vi "ScriptLoop.vi"   [LabVIEW 2012]
types:
  T1 = cluster{"Name":string, "Parameters":string[], "Start Conditional":cluster{"String":string, "avgs":cluster{"Expression":string, "Durration":dbl, "Replacement":string, "Values":dbl[]}[]}, "End Conditional":cluster{"String":string, "avgs":cluster{"Expression":string, "Durration":dbl, "Replacement":string, "Values":dbl[]}[]}, "Running":bool}
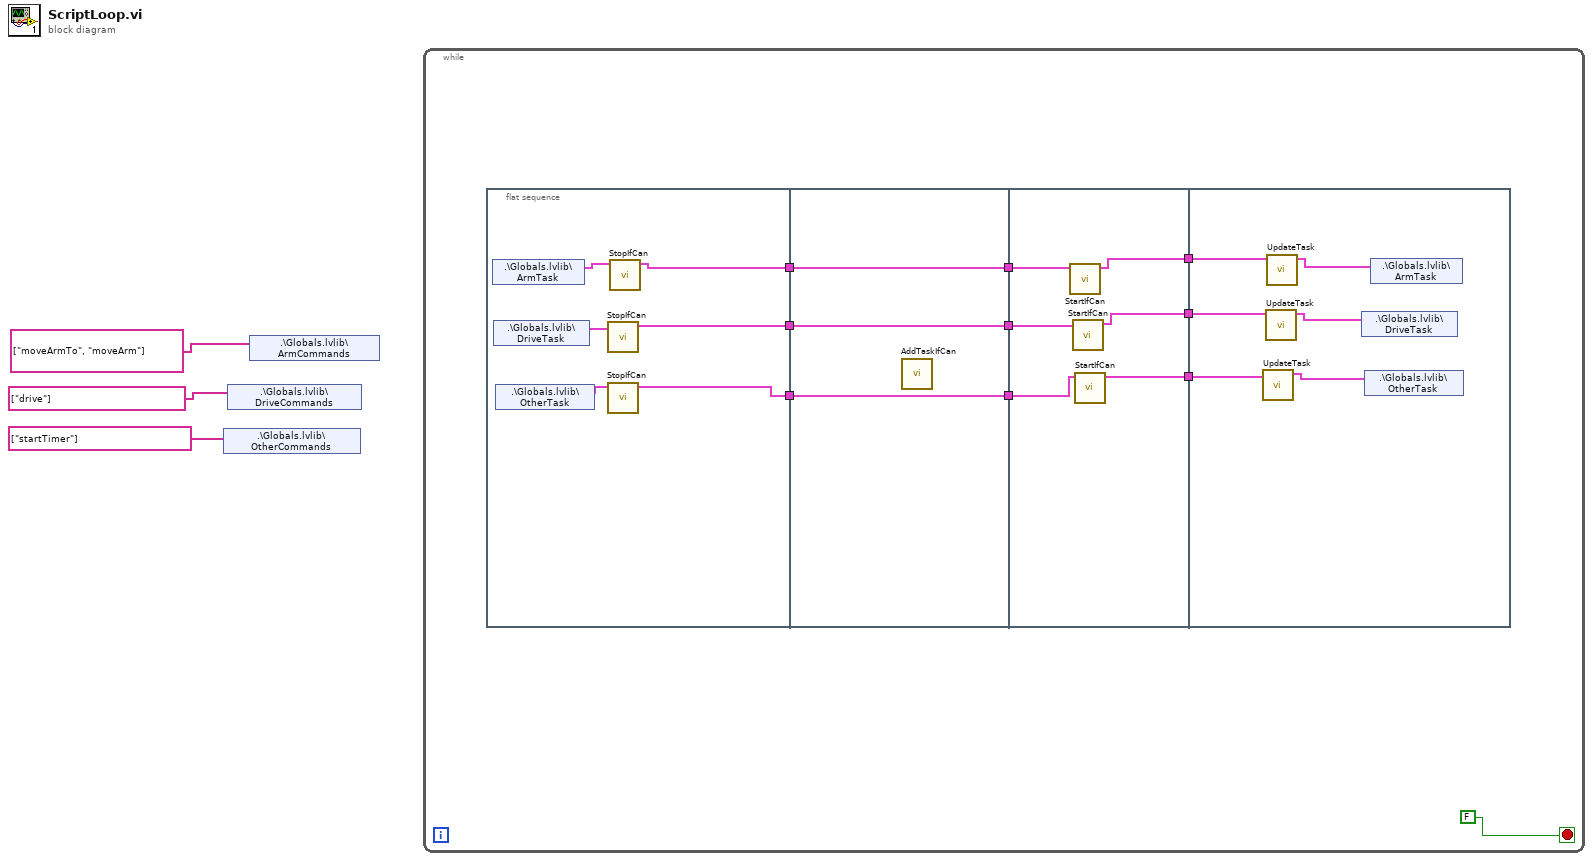
[diagram p0: block diagram]
diagram:
  n1 = shared-variable ".\\Globals.lvlib\\OtherCommands"(string[] ["startTimer"]) -> ()  [unwired: 1 in, 1 out]
  n2 = shared-variable ".\\Globals.lvlib\\DriveCommands"(string[] ["drive"]) -> ()  [unwired: 1 in, 1 out]
  n3 = shared-variable ".\\Globals.lvlib\\ArmCommands"(string[] ["moveArmTo", "moveArm"]) -> ()  [unwired: 1 in, 1 out]
  n4 = while {
    stop <- FALSE stop-if-true
    n5 = flat-sequence {
      tunnel: [w16] -> w13
      tunnel: [w15] -> w10
      tunnel: [w14] -> w8
      tunnel: w13 -> [w22]
      tunnel: [w22] -> w12
      tunnel: [w21] -> w11
      tunnel: w10 -> [w21]
      tunnel: [w20] -> w9
      tunnel: w8 -> [w20]
      tunnel: w12 -> [w28]
      tunnel: w11 -> [w27]
      tunnel: w9 -> [w26]
      tunnel: [w25] -> w7
      tunnel: [w24] -> w6
      tunnel: [w23] -> w5
      tunnel: w7 -> [w34]
      tunnel: w6 -> [w33]
      tunnel: w5 -> [w32]
      frame #0 {
        n6 = shared-variable ".\\Globals.lvlib\\ArmTask"() -> (w17:T1)  [unwired: 1 in, 1 out]
        n7 = shared-variable ".\\Globals.lvlib\\DriveTask"() -> (w19:T1)  [unwired: 1 in, 1 out]
        n8 = shared-variable ".\\Globals.lvlib\\OtherTask"() -> (w18:T1)  [unwired: 1 in, 1 out]
        n9 = call "StopIfCan.vi"("In Task"=w19) -> ("Out Task"=w15:T1)  [unwired: 10 in]
        n10 = call "StopIfCan.vi"("In Task"=w18) -> ("Out Task"=w16:T1)  [unwired: 10 in]
        n11 = call "StopIfCan.vi"("In Task"=w17) -> ("Out Task"=w14:T1)  [unwired: 10 in]
      }
      frame #1 {
        n12 = call "AddTaskIfCan.vi"() -> ()  [unwired: 12 in]
      }
      frame #2 {
        n13 = call "StartIfCan.vi"("In Task"=w26) -> ("Out Task"=w25:T1)  [unwired: 10 in]
        n14 = call "StartIfCan.vi"("In Task"=w27) -> ("Out Task"=w24:T1)  [unwired: 10 in]
        n15 = call "StartIfCan.vi"("In Task"=w28) -> ("Out Task"=w23:T1)  [unwired: 10 in]
      }
      frame #3 {
        n16 = call "UpdateTask.vi"("Task In"=w32) -> ("Task Out"=w31:T1)  [unwired: 10 in]
        n17 = call "UpdateTask.vi"("Task In"=w33) -> ("Task Out"=w30:T1)  [unwired: 10 in]
        n18 = call "UpdateTask.vi"("Task In"=w34) -> ("Task Out"=w29:T1)  [unwired: 10 in]
        n19 = shared-variable ".\\Globals.lvlib\\DriveTask"(w30) -> ()  [unwired: 1 in, 1 out]
        n20 = shared-variable ".\\Globals.lvlib\\OtherTask"(w31) -> ()  [unwired: 1 in, 1 out]
        n21 = shared-variable ".\\Globals.lvlib\\ArmTask"(w29) -> ()  [unwired: 1 in, 1 out]
      }
    }
  }
